vi "Teardown Examples SCD.vi"(8 "error in (no error)":errorcluster, 11 "Monochromator in":refnum<class "SCD.lvclass">) -> (0 "error out":errorcluster)   [LabVIEW 2020, in "Examples.lvlib"]
doc: "Closes the connection to all connected devices and closes the ICL."
uses:
  Examples.lvlib
  Classes/SCD/SCD.lvclass
  Classes/DeviceManager/DeviceManager.lvlib
panel:
  # "Connector Pane"
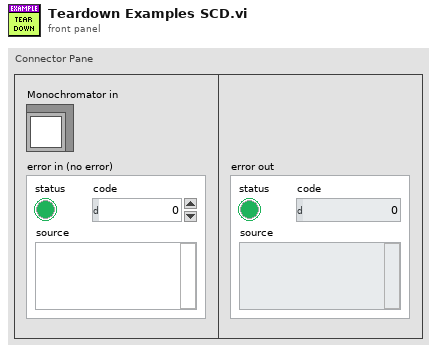
[diagram p1: front panel]
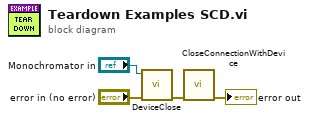
[diagram p0: block diagram]
diagram:
  n1 = call-dynamic "DeviceClose.vi"("error in (no error)"="error in (no error)", "SCD in"="Monochromator in") -> ("error out"=w2:errorcluster)  [unwired: 5 in, 4 out]
  n2 = call "CloseConnectionWithDevice.vi"("error in (no error)"=w2) -> ("error out"=→"error out":errorcluster)  [unwired: 10 in]
